vi "configCNT.vi"(8 "error in (no error)":errorcluster, 10 "Channel  1":i32(ring) items=["A", "B"]) -> (0 "error out":errorcluster, 3 "CNT90 out":refnum<class "CNT90.lvclass">)   [LabVIEW 2019, in "CNT90.lvclass"]
uses:
  CNT90.lvclass
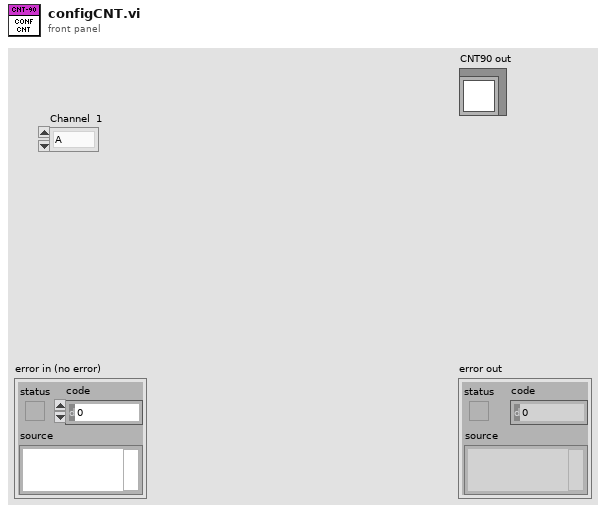
[diagram p1: front panel]
types:
  T1 = cluster{"error":bool, "code":i32, "source":string}
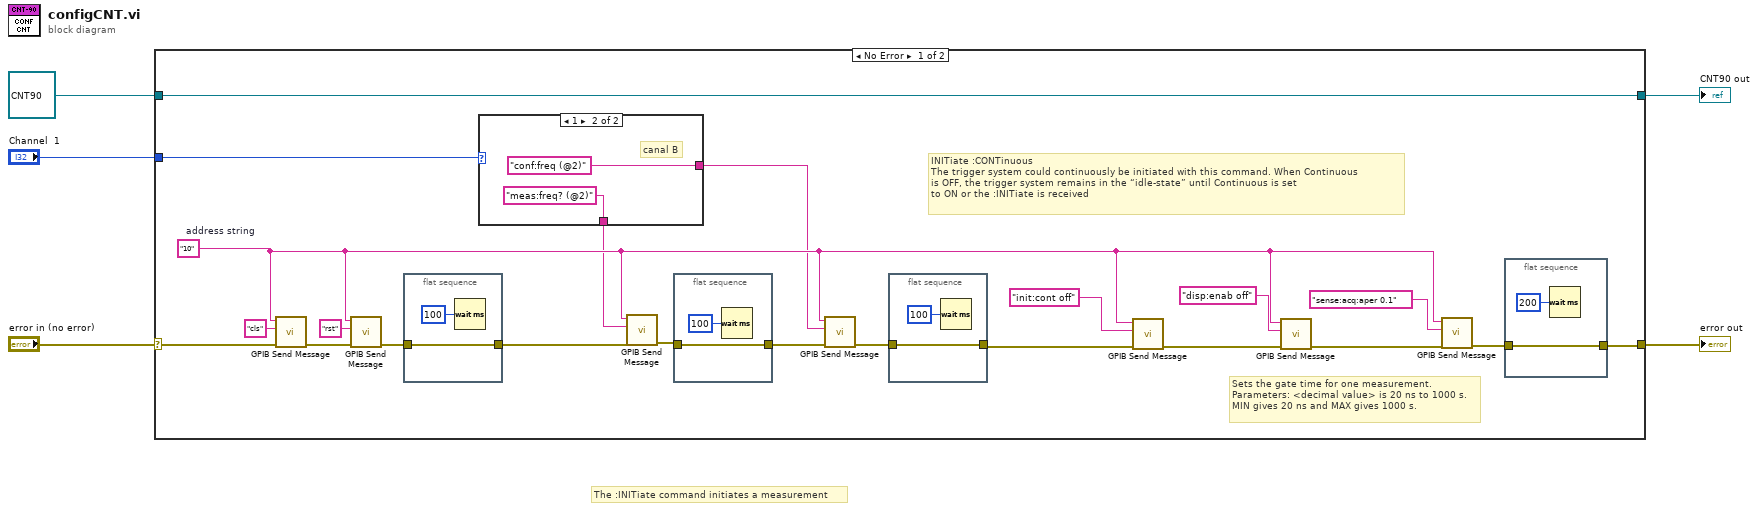
[diagram p0: block diagram]
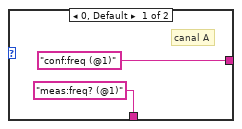
[diagram p2: hidden frame]
diagram:
  # "The :INITiate command initiates a measurement"
  n1 = case shown="No Error" "error in (no error)" {
    selector: "error in (no error)" -> [w11 w41]
    tunnel: [w10 w41] -> w4
    tunnel: [w9 w40] -> w2
    tunnel: refnum<class "CNT90.lvclass"> refnum ("CNT90 in") -> [w9 w40]
    tunnel: "Channel  1" -> [w8 _]
    frame No Error {
      w17 = "10"  # address string
      # "Sets the gate time for one measurement.\nParameters: <decimal value> is 20 ns to 1000 s.\nMIN gives 20 ns and MAX gives 1000 s."
      # "INITiate :CONTinuous\nThe trigger system could continuously be initiated with this command. When Continuous\nis OFF, the trigger system remains in the “idle-state” until Continuous is set\nto ON or the :INITiate is received"
      n2 = call <instrlib>:"GPIB Send Message.vi"("address string"=w17, "write buffer"="cls", "error in"=w11) -> ("error out"=w25:T1)  [unwired: 4 in, 2 out]
      n3 = call <instrlib>:"GPIB Send Message.vi"("address string"=w17, "write buffer"="rst", "error in"=w25) -> ("error out"=w23:T1)  [unwired: 4 in, 2 out]
      n4 = flat-sequence {
        tunnel: [w37] -> w24
        tunnel: w23 -> [w37]
        frame #0 {
          n5 = Wait (ms)(milliseconds to wait=u32 100) -> ()  [unwired: 1 out]
        }
      }
      n6 = case shown="1" w8 {
        tunnel: ["conf:freq (@1)" ("write buffer") "conf:freq (@2)" ("write buffer")] -> w7
        tunnel: ["meas:freq? (@1)" ("write buffer") "meas:freq? (@2)" ("write buffer")] -> w6
        frame 0, Default {
          # "canal A"
        }
        frame 1 {
          # "canal B"
        }
      }
      n7 = call <instrlib>:"GPIB Send Message.vi"("address string"=w17, "write buffer"=w6, "error in"=w24) -> ("error out"=w22:T1)  [unwired: 4 in, 2 out]
      n8 = flat-sequence {
        tunnel: [w35] -> w21
        tunnel: w22 -> [w35]
        frame #0 {
          n9 = Wait (ms)(milliseconds to wait=u32 100) -> ()  [unwired: 1 out]
        }
      }
      n10 = call <instrlib>:"GPIB Send Message.vi"("address string"=w17, "write buffer"=w7, "error in"=w21) -> ("error out"=w20:T1)  [unwired: 4 in, 2 out]
      n11 = flat-sequence {
        tunnel: [w33] -> w19
        tunnel: w20 -> [w33]
        frame #0 {
          n12 = Wait (ms)(milliseconds to wait=u32 100) -> ()  [unwired: 1 out]
        }
      }
      n13 = call <instrlib>:"GPIB Send Message.vi"("address string"=w17, "write buffer"="init:cont off", "error in"=w19) -> ("error out"=w18:T1)  [unwired: 4 in, 2 out]
      n14 = call <instrlib>:"GPIB Send Message.vi"("address string"=w17, "write buffer"="disp:enab off", "error in"=w18) -> ("error out"=w27:T1)  [unwired: 4 in, 2 out]
      n15 = call <instrlib>:"GPIB Send Message.vi"("address string"=w17, "write buffer"="sense:acq:aper 0.1", "error in"=w27) -> ("error out"=w26:T1)  [unwired: 4 in, 2 out]
      n16 = flat-sequence {
        tunnel: [w39] -> w10
        tunnel: w26 -> [w39]
        frame #0 {
          n17 = Wait (ms)(milliseconds to wait=u32 200) -> ()  [unwired: 1 out]
        }
      }
    }
    frame Error {
    }
  }
  "error out" <- w4
  "CNT90 out" <- w2
